vi "auto.vi"   [LabVIEW 2014, in "Janga.lvrbt"]
uses:
  Janga.lvrbt
  <vilib>/NXT/Block Support/NXT_OutputPort.ctl
  <vilib>/NXT/NXTIO Xnodes/NXTIONodeSubVIs/NXTMotorRunDistance.vi
  <vilib>/NXT/NXTIO Xnodes/NXTIONodeSubVIs/LEGOStopAllMotors.vi
  <vilib>/NXT/Subs/LVHSConnector.ctl
  <vilib>/NXT/NXTIO Xnodes/AddressXNode/NXTIOAddress.xnode
  <vilib>/NXT/NXTIO Xnodes/NXTIOXNode/NXTIO.xnode
  <vilib>/NXT/LegoClasses/BrickReference/BrickReference.lvclass
  <vilib>/NXT/NXTIO Xnodes/NXTIONodeSubVIs/NXTStopMotors.vi
types:
  T1 = typedef "NXT_OutputPort.ctl" = u8
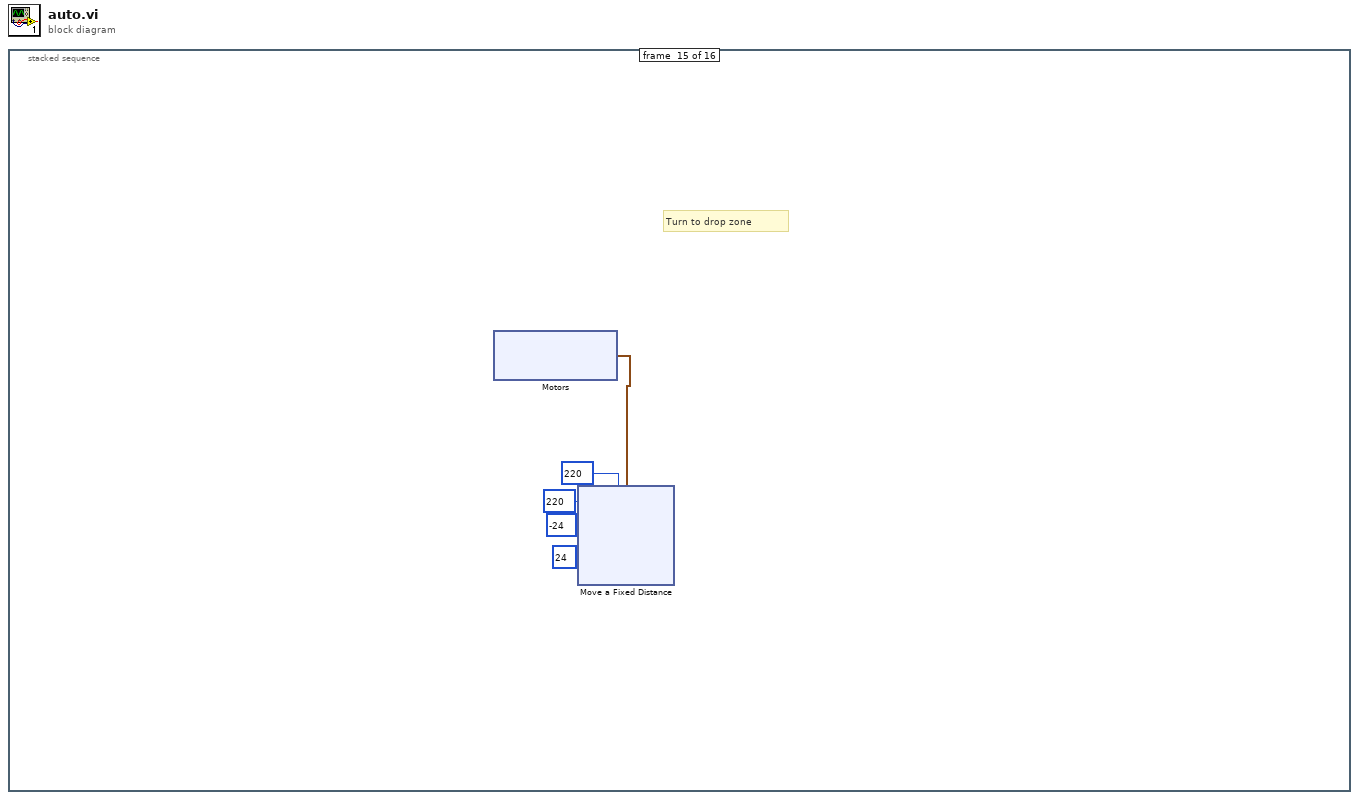
[diagram p0: block diagram]
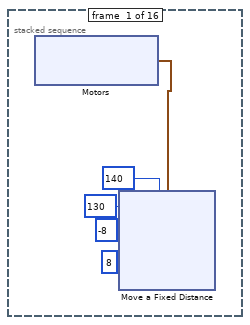
[diagram p2: hidden frame]
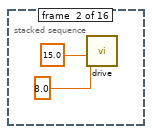
[diagram p3: hidden frame]
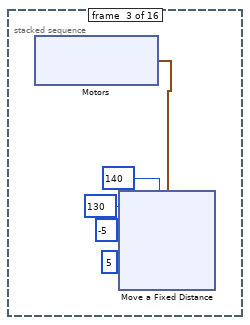
[diagram p4: hidden frame]
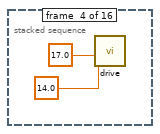
[diagram p5: hidden frame]
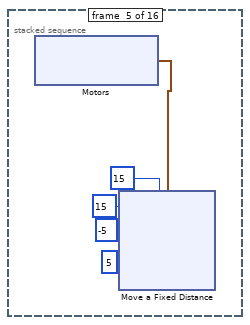
[diagram p6: hidden frame]
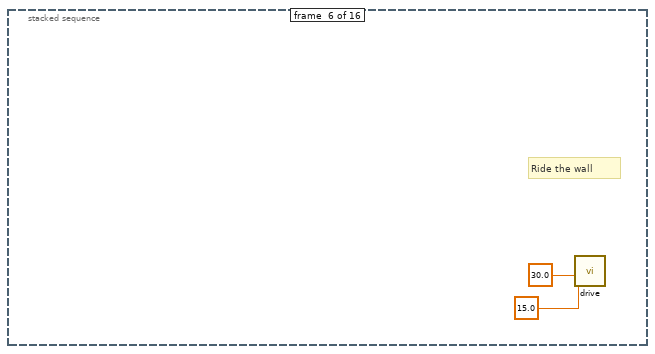
[diagram p7: hidden frame]
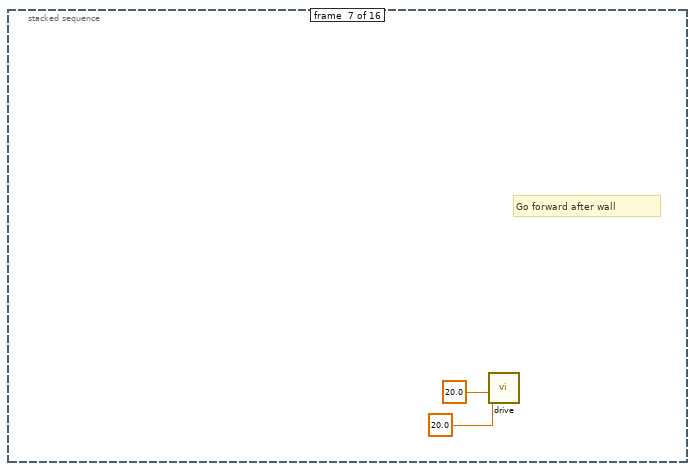
[diagram p8: hidden frame]
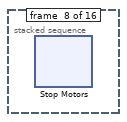
[diagram p9: hidden frame]
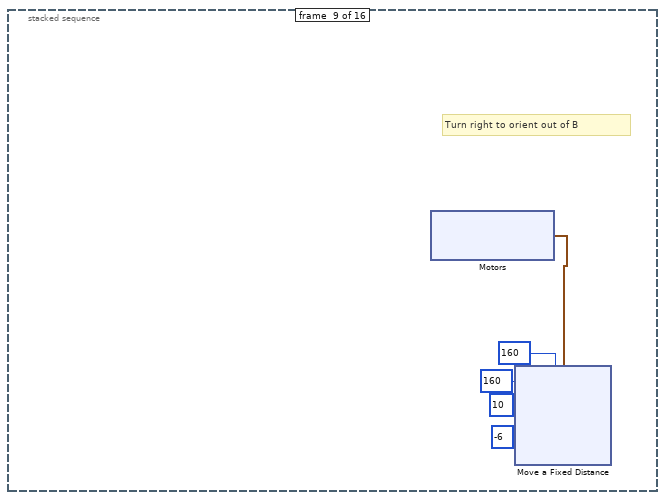
[diagram p10: hidden frame]
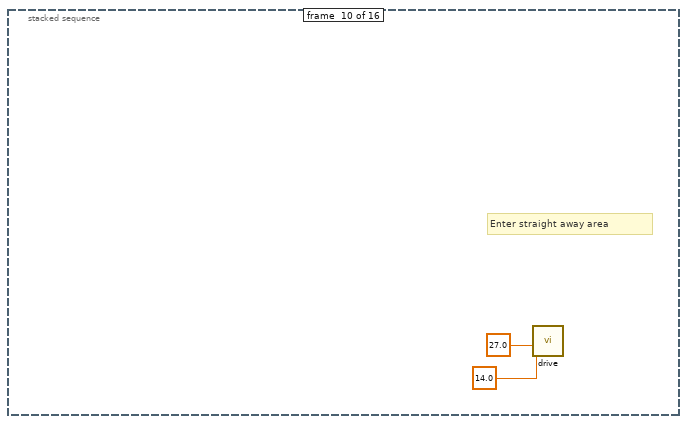
[diagram p11: hidden frame]
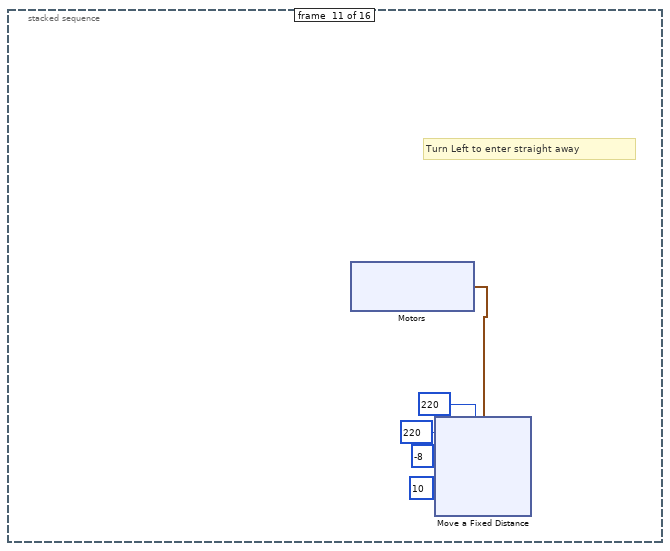
[diagram p12: hidden frame]
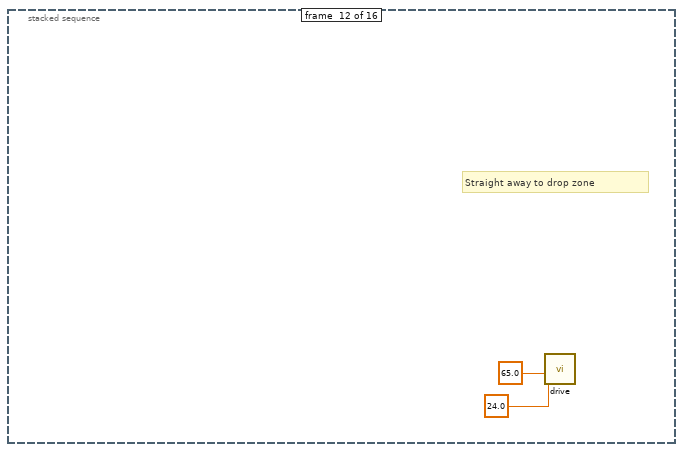
[diagram p13: hidden frame]
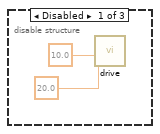
[diagram p15: hidden frame]
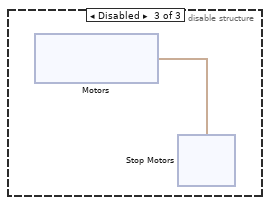
[diagram p16: hidden frame]
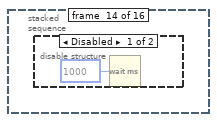
[diagram p17: hidden frame]
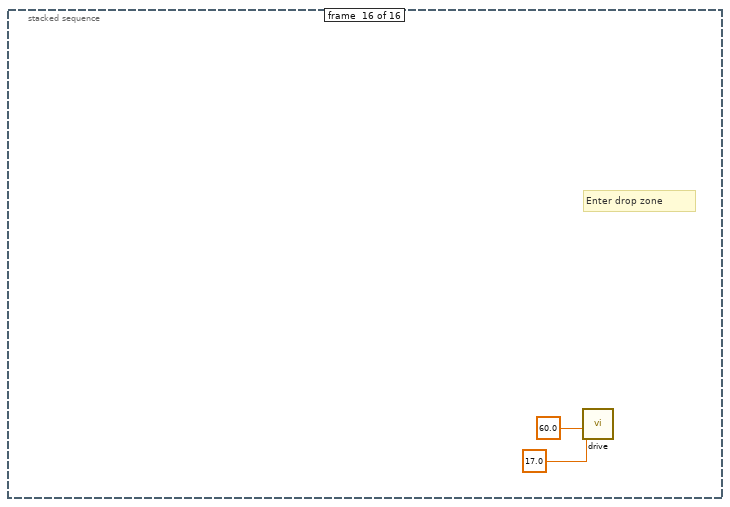
[diagram p19: hidden frame]
diagram:
  n1 = stacked-sequence {
    frame #0 {
      n2 = xnode "Motors"() -> ("Motor"=w5:cluster{"Port":T1, "Port":T1})
      n3 = xnode "Move a Fixed Distance"("Speed 2"=i8 8, "Speed 1"=i8 -8, "Distance 2"=130, "Distance 1"=140, "Motors"=w5) -> ()  [unwired: 1 in, 1 out]
    }
    frame #1 {
      n4 = call "drive.vi"("Speed"=8.0, "Distance (cm)"=15.0) -> ()  [unwired: 10 in]
    }
    frame #2 {
      n5 = xnode "Motors"() -> ("Motor"=w25:cluster{"Port":T1, "Port":T1})
      n6 = xnode "Move a Fixed Distance"("Speed 2"=i8 5, "Speed 1"=i8 -5, "Distance 2"=130, "Distance 1"=140, "Motors"=w25) -> ()  [unwired: 1 in, 1 out]
    }
    frame #3 {
      n7 = call "drive.vi"("Speed"=14.0, "Distance (cm)"=17.0) -> ()  [unwired: 10 in]
    }
    frame #4 {
      n8 = xnode "Motors"() -> ("Motor"=w45:cluster{"Port":T1, "Port":T1})
      n9 = xnode "Move a Fixed Distance"("Speed 2"=i8 5, "Speed 1"=i8 -5, "Distance 2"=15, "Distance 1"=15, "Motors"=w45) -> ()  [unwired: 1 in, 1 out]
    }
    frame #5 {
      # "Ride the wall"
      n10 = call "drive.vi"("Speed"=15.0, "Distance (cm)"=30.0) -> ()  [unwired: 10 in]
    }
    frame #6 {
      # "Go forward after wall"
      n11 = call "drive.vi"("Speed"=20.0, "Distance (cm)"=20.0) -> ()  [unwired: 10 in]
    }
    frame #7 {
      n12 = xnode "Stop Motors"() -> ()  [unwired: 2 in, 1 out]
    }
    frame #8 {
      # "Turn right to orient out of B"
      n13 = xnode "Motors"() -> ("Motor"=w72:cluster{"Port":T1, "Port":T1})
      n14 = xnode "Move a Fixed Distance"("Speed 2"=i8 -6, "Speed 1"=i8 10, "Distance 2"=160, "Distance 1"=160, "Motors"=w72) -> ()  [unwired: 1 in, 1 out]
    }
    frame #9 {
      # "Enter straight away area"
      n15 = call "drive.vi"("Speed"=14.0, "Distance (cm)"=27.0) -> ()  [unwired: 10 in]
    }
    frame #10 {
      # "Turn Left to enter straight away"
      n16 = xnode "Motors"() -> ("Motor"=w92:cluster{"Port":T1, "Port":T1})
      n17 = xnode "Move a Fixed Distance"("Speed 2"=i8 10, "Speed 1"=i8 -8, "Distance 2"=220, "Distance 1"=220, "Motors"=w92) -> ()  [unwired: 1 in, 1 out]
    }
    frame #11 {
      # "Straight away to drop zone"
      n18 = call "drive.vi"("Speed"=24.0, "Distance (cm)"=65.0) -> ()  [unwired: 10 in]
    }
    frame #12 {
      # "Slow down straight away"
      n19 = disable-structure shown="Enabled" {
        frame Disabled {
          n20 = call "drive.vi"("Speed"=20.0, "Distance (cm)"=10.0) -> ()  [unwired: 10 in]
        }
        frame Enabled {
        }
        frame Disabled {
          n21 = xnode "Motors"() -> ("Motor"=w110:cluster{"Port":T1, "Port":T1})
          n22 = xnode "Stop Motors"("Motors"=w110) -> ()  [unwired: 1 in, 1 out]
        }
      }
    }
    frame #13 {
      n23 = disable-structure shown="Disabled" {
        frame Disabled {
          n24 = Wait (ms)(milliseconds to wait=u32 1000) -> ()  [unwired: 1 out]
        }
        frame Enabled {
        }
      }
    }
    frame #14 {
      # "Turn to drop zone"
      n25 = xnode "Motors"() -> ("Motor"=w122:cluster{"Port":T1, "Port":T1})
      n26 = xnode "Move a Fixed Distance"("Speed 2"=i8 24, "Speed 1"=i8 -24, "Distance 2"=220, "Distance 1"=220, "Motors"=w122) -> ()  [unwired: 1 in, 1 out]
    }
    frame #15 {
      # "Enter drop zone"
      n27 = call "drive.vi"("Speed"=17.0, "Distance (cm)"=60.0) -> ()  [unwired: 10 in]
    }
  }
